vi "writeLogMessage.vi"(8 "error in (no error)":errorcluster, 10 "WriteLogMessageInput":T1, 11 "CSVTestLog in":refnum<class "CSVTestLog.lvclass">) -> (0 "error out":errorcluster, 3 "CSVTestLog out":refnum<class "CSVTestLog.lvclass">)   [LabVIEW 2015, in "CSVTestLog.lvclass"]
uses:
  CSVTestLog.lvclass
  Typedefs/WriteLogMessageInput.ctl
  Typedefs/TestScenarioTypes.ctl
  Typedefs/PassFailTest.ctl
  CSVTestLog.lvclass/CSVTestLog.ctl
  Typedefs/ILCBTTypedefs.lvlib
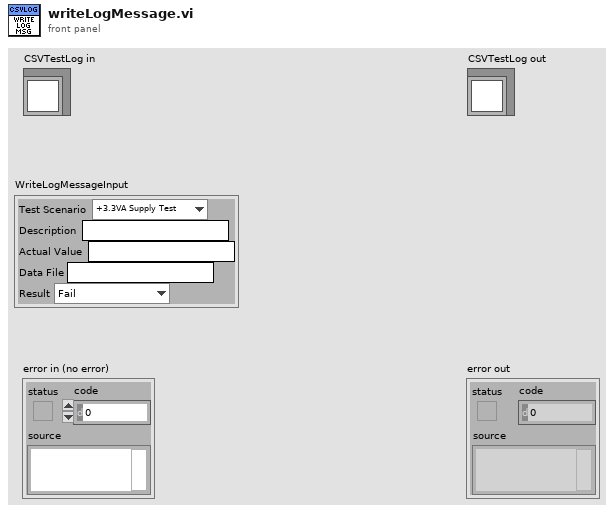
[diagram p1: front panel]
types:
  T1 = typedef "ILCBTTypedefs.lvlib/WriteLogMessageInput.ctl" = cluster{"Test Scenario":T2, "Description":string, "Actual Value":string, "Data File":string, "Result":T3}
  T2 = typedef "ILCBTTypedefs.lvlib/TestScenarioTypes.ctl" = enum16{"+3.3VA Supply Test", "+3.3VD Supply Test", "+5VA Supply Test", "+5VD Supply Test", "Unique ID Test", "TEDS Status Test", "LIMSW1_TTL Low Test", "LIMSW1_TTL High Test", "LIMSW2_TTL Low Test", "LIMSW2_TTL High Test", "Tachometer Low Test", "Tachometer High Test", "SSR_TTL Low Test", "SSR_TTL High Test", "SM_GPI Low Test", "SM_GPI High Test", "CW Motion Without Limit Test", "CW Motion With Limit Test", "CW Motion With Both Limits Test", "CW Motion on CCW Limit Test", "CCW Motion Without Limit Test", "CCW Motion With Limit Test", "CCW Motion With Both Limits Test", "CCW Motion on CW Limit Test", "RS232-TXD Low Test", "RS232-TXD High Test", "RS232-RTS Low Test", "RS232-RTS High Test", "RS232-RXD Low Test", "RS232-RXD High Test", "RS232-CTS Low Test", "RS232-CTS High Test", "Out_SS Low Test", "Out_SS High Test", "Out_SDI Low Test", "Out_SDI High Test", "Out_SCLK Low Test", "Out_SCLK High Test", "Reset Low Test", "Reset High Test", "1 Channel ADC Test", "3 Channel ADC Test", "5 Channel ADC Test", "Vref Test", "ROT Test", "DAC1 Test", "DAC2 Test", "DAC3 Test", "DAC4 Test", "BIAS Test", "EXC1 Test", "EXC2 Test", "EXC3 Test", "EXC4 Test"}
  T3 = typedef "ILCBTTypedefs.lvlib/PassFailTest.ctl" = enum16{"Fail", "Pass", "NA"}
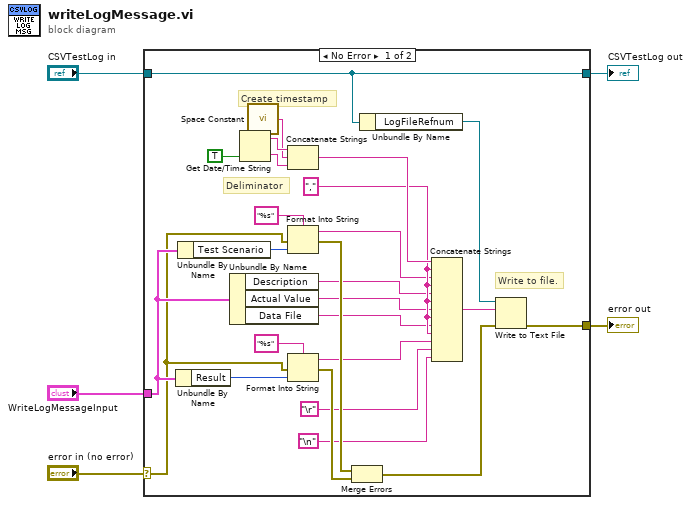
[diagram p0: block diagram]
diagram:
  n1 = case shown="No Error" "error in (no error)" {
    selector: "error in (no error)" -> [w17 w32]
    tunnel: "CSVTestLog in" -> [w31 w33]
    tunnel: [w31 w33] -> w3
    tunnel: "WriteLogMessageInput" -> [w24 _]
    tunnel: [w25 w32] -> w1
    frame No Error {
      w15 = ","
      # "Write to file."
      # "Deliminator"
      # "Create timestamp"
      n2 = Unbundle By Name(w24) -> ("Result"=w22:T3)
      n3 = Unbundle By Name(w24) -> ("Test Scenario"=w23:T2)
      n4 = Unbundle By Name(w24) -> ("Description"=w13:string, "Actual Value"=w12:string, "Data File"=w11:string)
      n5 = Get Date/Time String(want seconds? (F)=TRUE) -> (date string=w28:string, time string=w27:string)  [unwired: 2 in]
      n6 = call <vilib>:"Space Constant.vi"() -> ("String"=w26:string)
      n7 = Concatenate Strings(w28, w26, w27) -> (w16:string)
      n8 = Format Into String(format string="%s", error in=w17, w23) -> (resulting string=w14:string, error out=w19:errorcluster)  [unwired: 1 in]
      n9 = Format Into String(format string="%s", error in=w17, w22) -> (resulting string=w10:string, error out=w18:errorcluster)  [unwired: 1 in]
      n10 = Merge Errors(w19, w18) -> (w7:errorcluster)
      n11 = Unbundle By Name(w31) -> ("LogFileRefnum"=w30:refnum<file>)
      n12 = Concatenate Strings(w16, w15, w14, w15, w13, w15, w12, w15, w11, w15, w10, "\r", "\n") -> (w29:string)
      n13 = Write to Text File(file (use dialog)=w30, text=w29, error in=w7) -> (error out=w25:errorcluster)  [unwired: 1 in, 2 out]
    }
    frame Error {
    }
  }
  "error out" <- w1
  "CSVTestLog out" <- w3
